vi "ProdaNG.WabcoParts.Get.vi"(8 "error in (no error)":errorcluster, 11 "dbHandleIn":i32) -> (0 "error out":errorcluster, 2 "WabcoParts":T1[](array[typedef]), 3 "dbHandle":i32)   [LabVIEW 2016]
doc: "This function returns a product structure for a product, which is identified by a part and a serial number.\nImportant information: The field 'individual' was taken over from the field 'allgemein' of the legacy data directly. Because of this most products have the value 0 further on and only a few the value 1. \nParameter:\nhandle is an Integer, which is returned by the function Login() at the creation of a new connection.\nwabcoPartId is the Id of the part.\nserialNumber is the serial number of the product for the part above.\nproduct is a pointer on a product structure, which is filled if the returncode is 0. The structure must be defined in the calling program.\n\nReturncodes:\n0 No error\n< 0 ORACLE Error code\n6 (ERROR_INVALID_HANDLE) in case of an invalid handle\n1403 Record does not exist"
uses:
  Controls/ProdaNG.WabcoPart.ctl
  Controls/ProdaNG.WabcoPartSize.ctl
  <vilib>/Utility/importsl/GetValueByPointer/datatype.ctl
  <vilib>/Utility/importsl/GetValueByPointer/GetValueByPointer.xnode
  prodllNG.dll
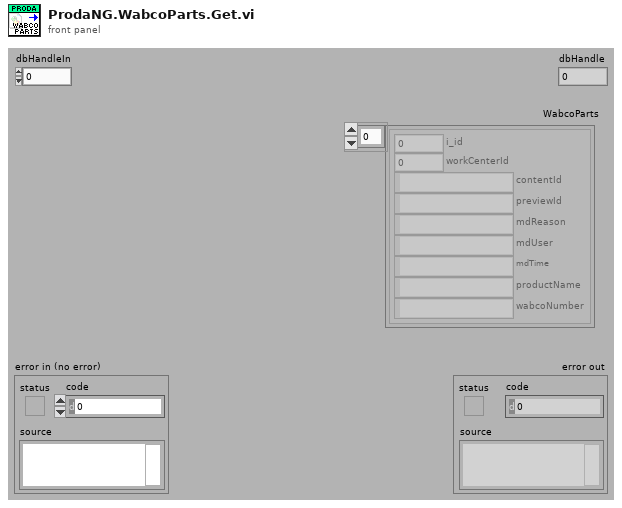
[diagram p1: front panel]
types:
  T1 = typedef "ProdaNG.WabcoPart.ctl" = cluster{"i_id":i32, "workCenterId":i32, "contentId":string, "previewId":string, "mdReason":string, "mdUser":string, "mdTime":string, "productName":string, "wabcoNumber":string}
  T2 = typedef "ProdaNG.WabcoPartSize.ctl" = cluster{"i_id":i32, "workCenterId":i32, "contentId":i32, "previewId":i32, "mdReason":i32, "mdUser":i32, "mdTime":i32, "productName":i32, "wabcoNumber":i32}
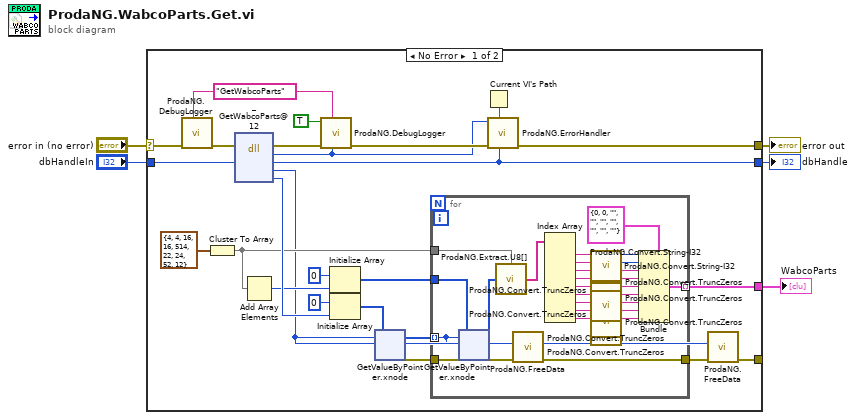
[diagram p0: block diagram]
diagram:
  n1 = case shown="No Error" "error in (no error)" {
    selector: "error in (no error)" -> [w25 w90]
    tunnel: [w30 w90] -> w4
    tunnel: "dbHandleIn" -> [w27 w89]
    tunnel: [w28 w89] -> w2
    tunnel: [w10 _] -> w1
    tunnel: [w7 _] -> _
    frame No Error {
      w21 = "GetWabcoParts" ("cmd")
      n2 = call "ProdaNG.DebugLogger.vi"("cmd"=w21, "error in (no error)"=w25) -> ("error out"=w24:errorcluster)  [unwired: 9 in]
      n3 = Cluster To Array(cluster=T2 {"i_id"=4, "workCenterId"=4, "contentId"=16, "previewId"=16, "mdReason"=514, "mdUser"=22, "mdTime"=24, "productName"=52, "wabcoNumber"=12} ("WabcoPart")) -> (array=w11:i32[])
      n4 = dll-call lib="D:/svn/LineTraceSystem/SOFTWARE/sources/Database/ProdaNG/prodllNG.dll" fn="_GetWabcoParts@12" ("ProDLL wrapper.dll:ProDLL_wrapper_GetWabcoParts_GetData")(error in=w24, "dbHandle"=w27) -> (error out=w23:errorcluster, "return type"=w20:i32, "dbHandle"=w28:i32, "wabcoPartsPtr"=w8:u32, "countPtr"=w15:i32)  [unwired: 4 in, 1 out]
      n5 = Add Array Elements(numeric array=w11) -> (sum=w12:i32)
      n6 = call "ProdaNG.DebugLogger.vi"("return type"=w20, "cmd"=w21, "error in (no error)"=w23, "done? (F)"=TRUE) -> ("error out"=w22:errorcluster)  [unwired: 7 in]
      n7 = Initialize Array(u8 0 ("element"), w12) -> (w13:u8[])
      n8 = Initialize Array(u32 0 ("element"), w15) -> (w19:u32[])
      n9 = xnode "GetValueByPointer.xnode"("Pointer"=w8, "InputType"=w19) -> ("Output"=w16:u32[], "ErrorOut"=w17:errorcluster)  [unwired: 2 in]
      n10 = for {
        tunnel: w17 -> [w58]
        tunnel: w16 -> [w40] mode=indexing
        tunnel: w13 -> [w57]
        tunnel: w11 -> [w46]
        tunnel: [w45] -> w10 mode=indexing
        tunnel: [w38] -> w9
        n11 = xnode "GetValueByPointer.xnode"("Pointer"=w40, "InputType"=w57, "ErrorIn"=w58) -> ("Output"=w48:u8[], "ErrorOut"=w39:errorcluster)  [unwired: 1 in]
        n12 = call "ProdaNG.Extract.U8[].vi"("unsigned byte array"=w48, "Sizes"=w46) -> ("Elements"=w47:string[])
        n13 = call "ProdaNG.FreeData.vi"("error in (no error)"=w39, "Pointers"=w40) -> ("error out"=w38:errorcluster)  [unwired: 9 in]
        n14 = Index Array(array=w47) -> (element #1=w50:string, element #2=w49:string, element #3=w35:string, element #4=w36:string, element #5=w54:string, element #6=w56:string, element #7=w44:string, element #8=w43:string, element #9=w31:string)  [unwired: 9 in]
        n15 = call "ProdaNG.Convert.String-I32.vi"("unsigned byte string"=w50) -> ("32bit integer"=w52:i32)  [unwired: 10 in]
        n16 = call "ProdaNG.Convert.String-I32.vi"("unsigned byte string"=w49) -> ("32bit integer"=w51:i32)  [unwired: 10 in]
        n17 = call "ProdaNG.Convert.TruncZeros.vi"("string with \\0s"=w35) -> ("LV string"=w34:string)  [unwired: 10 in]
        n18 = call "ProdaNG.Convert.TruncZeros.vi"("string with \\0s"=w36) -> ("LV string"=w33:string)  [unwired: 10 in]
        n19 = call "ProdaNG.Convert.TruncZeros.vi"("string with \\0s"=w54) -> ("LV string"=w53:string)  [unwired: 10 in]
        n20 = call "ProdaNG.Convert.TruncZeros.vi"("string with \\0s"=w56) -> ("LV string"=w55:string)  [unwired: 10 in]
        n21 = call "ProdaNG.Convert.TruncZeros.vi"("string with \\0s"=w44) -> ("LV string"=w42:string)  [unwired: 10 in]
        n22 = call "ProdaNG.Convert.TruncZeros.vi"("string with \\0s"=w43) -> ("LV string"=w41:string)  [unwired: 10 in]
        n23 = call "ProdaNG.Convert.TruncZeros.vi"("string with \\0s"=w31) -> ("LV string"=w32:string)  [unwired: 10 in]
        n24 = Bundle(cluster=T1 {"i_id"=0, "workCenterId"=0, "contentId"="", "previewId"="", "mdReason"="", "mdUser"="", "mdTime"="", "productName"="", "wabcoNumber"=""} ("WabcoPart"), "i_id"=w52, "workCenterId"=w51, "contentId"=w34, "previewId"=w33, "mdReason"=w53, "mdUser"=w55, "mdTime"=w42, "productName"=w41, "wabcoNumber"=w32) -> (w45:T1)
      }
      n25 = Current VI's Path() -> (path=w29:path)
      n26 = call "ProdaNG.ErrorHandler.vi"("dbHandleIn"=w28, "Path"=w29, "error in"=w22, "output_parameter"=w20) -> ("error out"=w30:errorcluster)  [unwired: 7 in]
      n27 = call "ProdaNG.FreeData.vi"("error in (no error)"=w9, "Pointers"=w8) -> ("error out"=w7:errorcluster)  [unwired: 9 in]
    }
    frame Error {
    }
  }
  "error out" <- w4
  "dbHandle" <- w2
  "WabcoParts" <- w1
